vi "Update AppInst Ring.vi"(8 "error in (no error)":errorcluster, 9 "Old Value":u16=65535, 10 "AppInst in":refnum<vi>, 11 "Ring in":refnum<vi>) -> (0 "error out":errorcluster, 1 "Selection Changed?":bool, 2 "AppInst out":refnum<vi>)   [LabVIEW 2013]
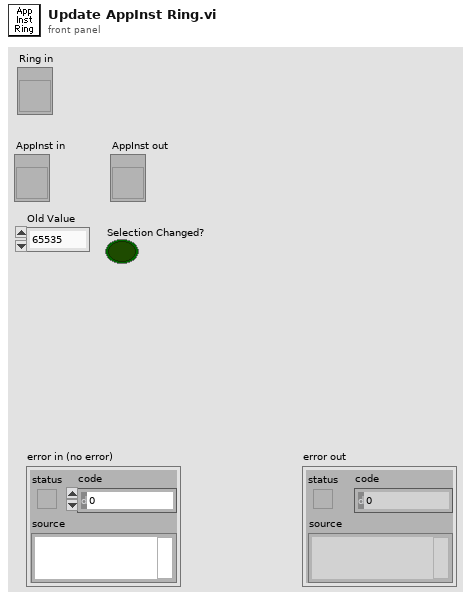
[diagram p1: front panel]
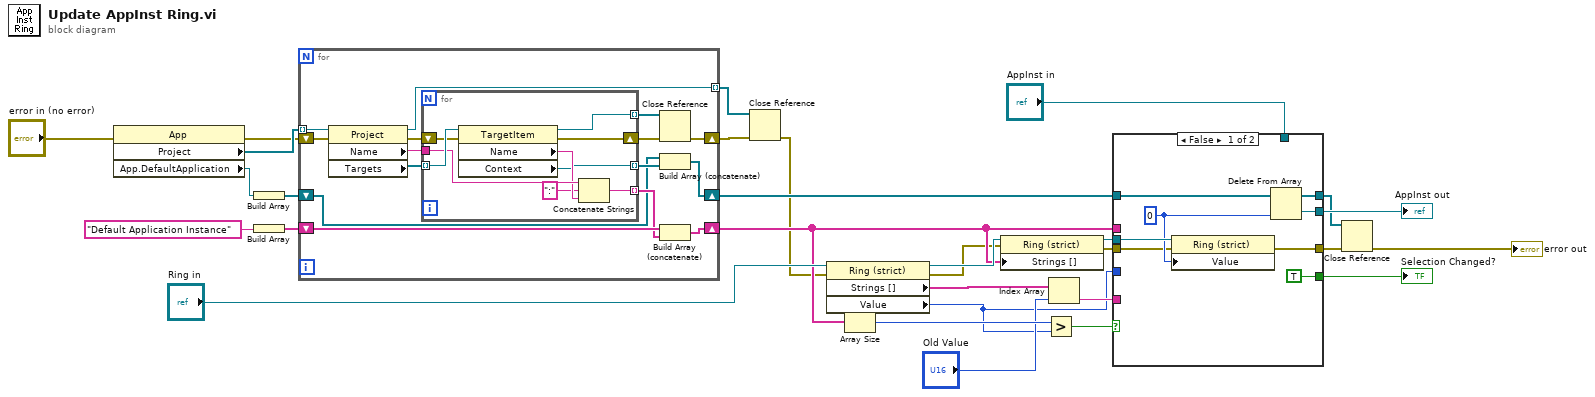
[diagram p0: block diagram]
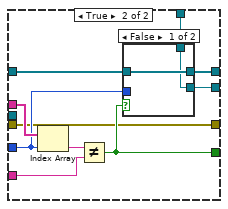
[diagram p2: hidden frame]
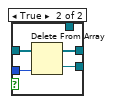
[diagram p3: hidden frame]
diagram:
  n1 = property class="App"(error in="error in (no error)") -> (error out=w28:errorcluster, "Project"=w29:refnum<vi>[], "App.DefaultApplication"=w10:refnum<vi>)  [unwired: 1 in, 1 out]
  n2 = Build Array(w10) -> (w26:refnum<vi>[])
  n3 = Build Array("Default Application Instance") -> (w27:string[])
  n4 = for {
    tunnel: w29 -> [w34] mode=indexing
    shift-right: [w40] -> w20
    shift-left: w27 -> [w42]
    shift-right: [w32] -> w14
    shift-left: w28 -> [w38]
    shift-right: [w36] -> w21
    shift-left: w26 -> [w35]
    tunnel: [w30] -> w13 mode=indexing
    n5 = property class="Project"(reference=w34, error in=w38) -> (reference out=w30:refnum<vi>, error out=w39:errorcluster, "Name"=w43:string, "Targets"=w44:refnum<vi>[])
    n6 = for {
      tunnel: w44 -> [w53] mode=indexing
      tunnel: w43 -> [w52]
      tunnel: [w49] -> w41 mode=indexing
      shift-right: [w46] -> w33
      shift-left: w39 -> [w48]
      tunnel: [w47] -> w37 mode=indexing
      tunnel: [w45] -> w31 mode=indexing
      n7 = property class="TargetItem"(reference=w53, error in=w48) -> (reference out=w45:refnum<vi>, error out=w46:errorcluster, "Name"=w51:string, "Context"=w47:refnum<vi>)
      n8 = Concatenate Strings(w52, ":" ("string"), w51) -> (w49:string)
    }
    n9 = Close Reference(reference=w31, error in (no error)=w33) -> (error out=w32:errorcluster)
    n10 = Build Array (concatenate)(w35, w37) -> (w36:refnum<vi>[])
    n11 = Build Array (concatenate)(w42, w41) -> (w40:string[])
  }
  n12 = Close Reference(reference=w13, error in (no error)=w14) -> (error out=w5:errorcluster)
  n13 = property class="Ring (strict)"(reference="Ring in", error in=w5) -> (reference out=w23:refnum<vi>, error out=w4:errorcluster, "Strings []"=w24:string[], "Value"=w7:u16)
  n14 = Array Size(array=w20) -> (size(s)=w19:i32)
  n15 = property class="Ring (strict)"(reference=w23, error in=w4, "Strings []"=w20) -> (reference out=w17:refnum<vi>, error out=w3:errorcluster)
  n16 = Greater?(x=w19, y=w7) -> (0:w18:bool)
  n17 = Index Array(array=w24, index="Old Value") -> (element=w11:string)
  n18 = case shown="False" w18 {
    tunnel: w20 -> [_ w71]
    tunnel: [TRUE w65] -> w22
    tunnel: w21 -> [w60 w69]
    tunnel: w7 -> [_ w68]
    tunnel: [w58 w67] -> w16
    tunnel: [w59 w66] -> w15
    tunnel: w17 -> [w57 _]
    tunnel: "AppInst in" -> [_ w64]
    tunnel: w11 -> [_ w63]
    tunnel: w3 -> [w55 w62]
    tunnel: [w54 w62] -> w2
    frame False {
      w56 = 0 ("index")
      n19 = property class="Ring (strict)"(reference=w57, error in=w55, "Value"=w56) -> (error out=w54:errorcluster)  [unwired: 1 out]
      n20 = Delete From Array(array=w60, index=w56) -> (deleted portion=w58:refnum<vi>, array with subset deleted=w59:refnum<vi>[])  [unwired: 1 in]
    }
    frame True {
      n21 = Index Array(array=w71, index=w68) -> (element=w70:string)
      n22 = Not Equal?(x=w70, y=w63) -> (x != y?=w65:bool)
      n23 = case shown="False" w65 {
        tunnel: w69 -> [w73 w77]
        tunnel: w68 -> [_ w76]
        tunnel: [w72 w75] -> w67
        tunnel: [w73 w74] -> w66
        tunnel: w64 -> [w72 _]
        frame False {
        }
        frame True {
          n24 = Delete From Array(array=w77, index=w76) -> (deleted portion=w75:refnum<vi>, array with subset deleted=w74:refnum<vi>[])  [unwired: 1 in]
        }
      }
    }
  }
  "AppInst out" <- w16
  "Selection Changed?" <- w22
  n25 = Close Reference(reference=w15, error in (no error)=w2) -> (error out=→"error out":errorcluster)
